vi "Destroy to Known Hosts.vi"(8 "Error In":errorcluster, 10 "Known Host":refnum<class "Known Host.lvclass">, 11 "KnownHosts In":refnum<class "Known Hosts.lvclass">) -> (0 "Error Out":errorcluster, 3 "KnownHosts Out":refnum<class "Known Hosts.lvclass">)   [LabVIEW 2018, in "Toolkit.lvlib" / "Known Host.lvclass"]
uses:
  Known Host.lvclass
  Known Hosts/Known Hosts.lvclass
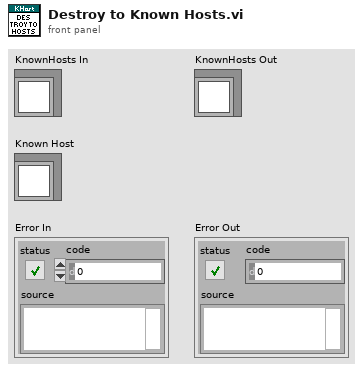
[diagram p1: front panel]
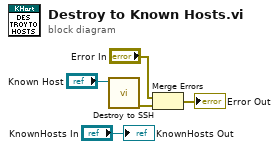
[diagram p0: block diagram]
diagram:
  n1 = call "Destroy to SSH.vi"("Known Host"="Known Host") -> ("Error Out"=w2:errorcluster)  [unwired: 9 in, 1 out]
  n2 = Merge Errors("Error In", w2) -> (→"Error Out":errorcluster)
  "KnownHosts Out" <- "KnownHosts In"
